vi "Create.vi"(8 "error in (no error)":errorcluster, 10 "Suite Name":string, 11 "LUnit Test Suite in":refnum<class "LUnit Test Suite.lvclass">) -> (0 "error out":errorcluster, 3 "LUnit Test Suite Out":refnum<class "LUnit Test Suite.lvclass">)   [LabVIEW 2020, in "LUnit Test Suite.lvclass"]
doc: "Initialize a test suite object."
uses:
  LUnit Test Suite.lvclass
  LUnit Test Suite.lvclass/LUnit Test Suite.ctl
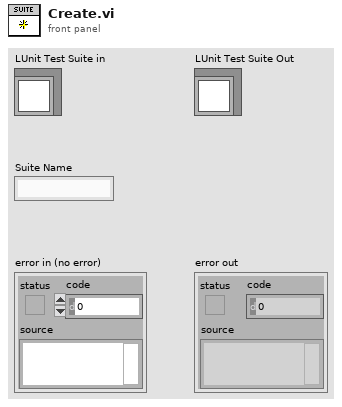
[diagram p1: front panel]
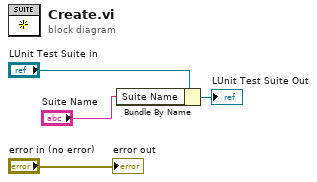
[diagram p0: block diagram]
diagram:
  n1 = Bundle By Name(cluster="LUnit Test Suite in", "Suite Name"="Suite Name") -> (→"LUnit Test Suite Out":refnum<class "LUnit Test Suite.lvclass">)
  "error out" <- "error in (no error)"
